vi "config db- FGV.vi"(8 "error in":errorcluster, 9 "Search string":string, 10 "Action":T1=enum."Write") -> (0 "error out":errorcluster, 2 "Found?":bool=TRUE)   [LabVIEW 2018, in "Controller.lvlib"]
doc: "Sends a message to all modules to abort and run shutdown code (with cleanup)."
uses:
  Controller.lvlib
  ctl/Config db action--enum.ctl
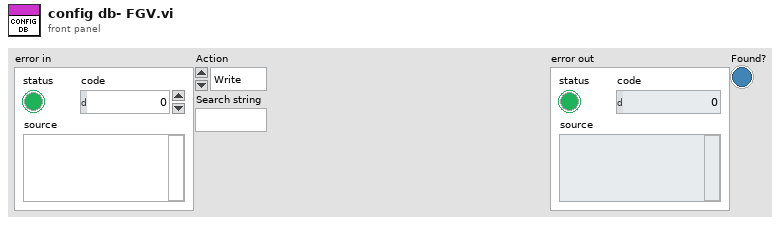
[diagram p1: front panel]
types:
  T1 = typedef "Controller.lvlib/Config db action--enum.ctl" = enum16{"Read", "Search", "Write"}
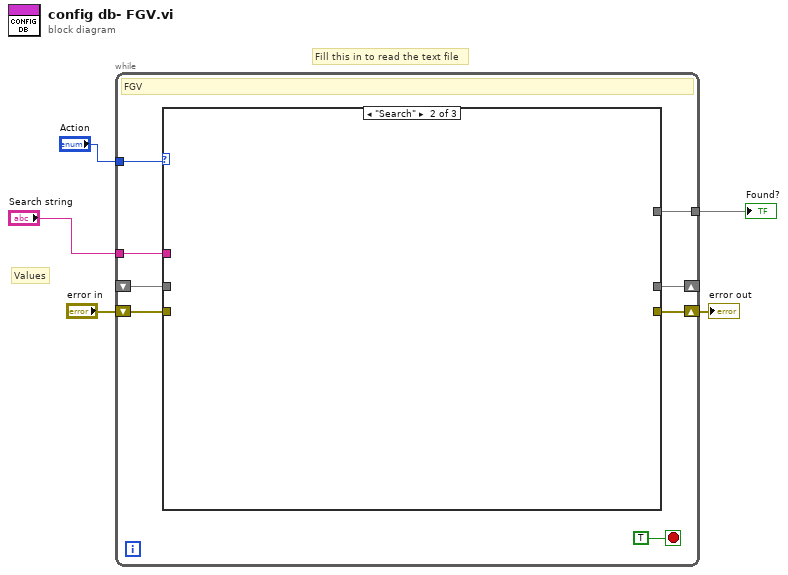
[diagram p0: block diagram]
diagram:
  # "Values"
  # "Fill this in to read the text file"
  n1 = while {
    tunnel: "Action" -> [w13]
    shift-right: [w11] -> _
    shift-left: _ -> [w10]
    shift-right: [w9] -> w3
    shift-left: "error in" -> [w8]
    tunnel: "Search string" -> [w7]
    tunnel: [w6] -> w1
    stop <- TRUE stop-if-true
    # "FGV"
    n2 = case shown="\"Search\"" w13 {
      tunnel: [w14 _ _] -> w11
      tunnel: w10 -> [w14 _ _]
      tunnel: [_ _ _] -> w9
      tunnel: w8 -> [_ _ _]
      tunnel: w7 -> [_ _ _]
      tunnel: [_ _ _] -> w6
      frame "Read" {
        # "T/F"
      }
      frame "Search" {
      }
      frame "Write" {
      }
    }
  }
  "error out" <- w3
  "Found?" <- w1
